vi "Camera Moving Test.vi"() -> ()   [LabVIEW 2017]
panel:
  out "Colour":T1(ring)=enum."None"
  out "Array":T2(array[ring])
  in  "stop":bool
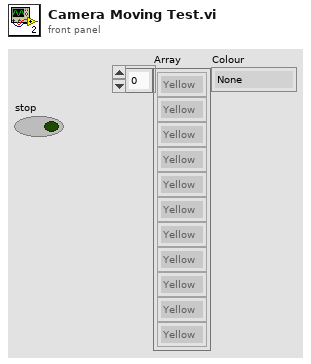
[diagram p1: front panel]
types:
  T1 = enum16{"Yellow", "Red", "Black", "Green", "None", "Black&Yellow"}
  T2 = enum16{"Yellow", "Red", "Black", "Green", "None", "Black&Yellow"}[]
  T3 = typedef "IMAQdx.ctl" = refnum<k21>
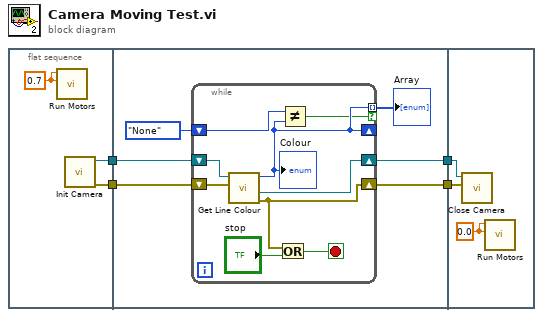
[diagram p0: block diagram]
diagram:
  n1 = flat-sequence {
    tunnel: [w6] -> w4
    tunnel: [w5] -> w3
    tunnel: w4 -> [w13]
    tunnel: w3 -> [w12]
    tunnel: [w11] -> w2
    tunnel: [w10] -> w1
    tunnel: w2 -> [w25]
    tunnel: w1 -> [w24]
    frame #0 {
      w7 = 0.7 ("Left motor speed (-1..1)")
      n2 = call "Run Motors.vi"("Right motor side (-1..1)"=w7, "Left motor speed (-1..1)"=w7) -> ()  [unwired: 10 in]
      n3 = call "Init Camera.vi"() -> ("error out 2"=w5:errorcluster, "session out"=w6:T3)  [unwired: 10 in]
    }
    frame #1 {
      n4 = while {
        shift-right: [w20] -> w11
        shift-left: w13 -> [w22]
        shift-right: [w18] -> w10
        shift-left: w12 -> [w21]
        shift-right: [w15] -> _
        shift-left: T1."None" ("Colour") -> [w16]
        tunnel: [w15] -> w8 mode=indexing if=w14
        stop <- w19 stop-if-true
        n5 = call "Get Line Colour.vi"("error out"=w21, "Session Out"=w22) -> ("error out 2"=w18:errorcluster, "Session Out 2"=w20:T3, "Colour"=w15:T1)  [unwired: 6 in, 1 out]
        "Colour" <- w15
        n6 = Or(x=w18, y="stop") -> (x .or. y?=w19:bool)
        n7 = Not Equal?(x=w16, y=w15) -> (x != y?=w14:bool)
      }
      "Array" <- w8
    }
    frame #2 {
      w23 = 0.0 ("Left motor speed (-1..1)")
      n8 = call "Close Camera.vi"("error in"=w24, "Session In"=w25) -> ()  [unwired: 8 in, 2 out]
      n9 = call "Run Motors.vi"("Right motor side (-1..1)"=w23, "Left motor speed (-1..1)"=w23) -> ()  [unwired: 10 in]
    }
  }
